vi "MainVI.vi"() -> ()   [LabVIEW 2020]
panel:
  in  "VOLUME (L)":dbl
  in  "FILL":bool
  in  "SET":bool
  in  "RE":bool
  in  "Down R":bool
  in  "R-L":bool
  in  "Up":bool
  in  "Hold":bool
  in  "Down":bool
  out "Boolean":bool
  out "Tank":dbl(slide) scale=0.0..100.0
  out "Boolean 2":bool
  # "EXTENDED BOTTLE SHIFTER"
  # "KUNAL KUMAR CHOUHAN"
  # "MALAVIYA NATIONAL INSTITUTE OF TECHNOLOGY"
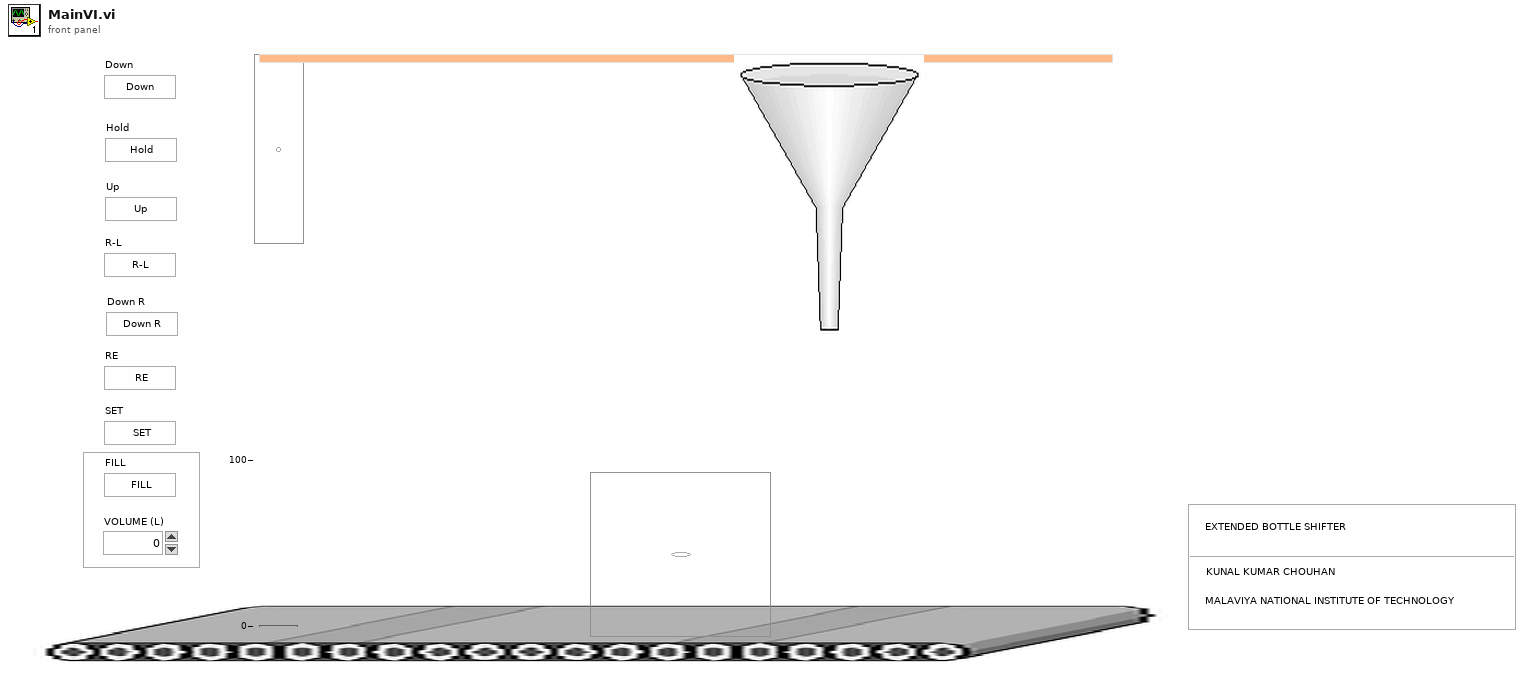
[diagram p1: front panel]
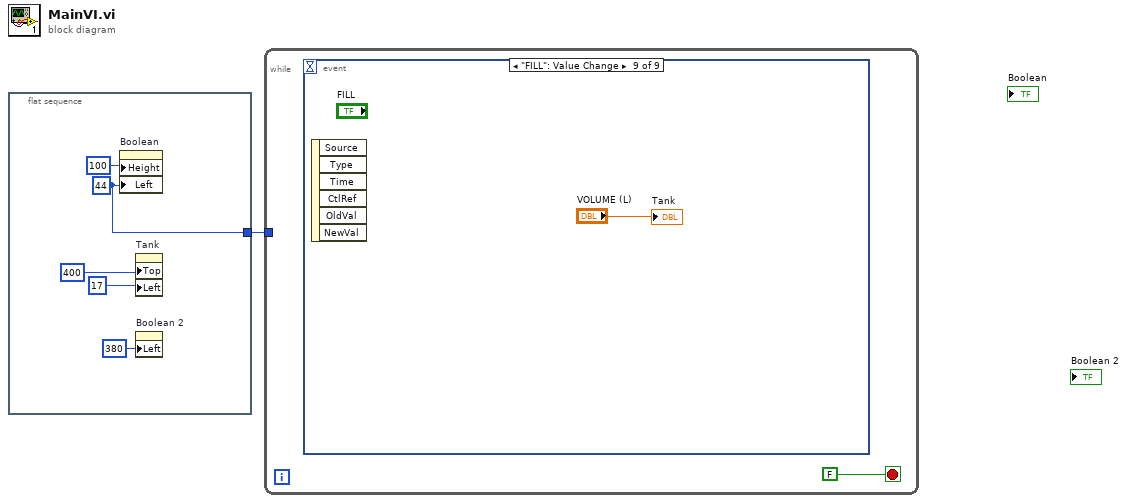
[diagram p0: block diagram]
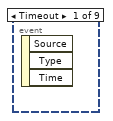
[diagram p2: hidden frame]
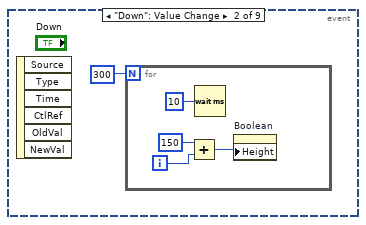
[diagram p3: hidden frame]
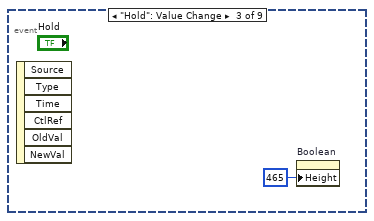
[diagram p4: hidden frame]
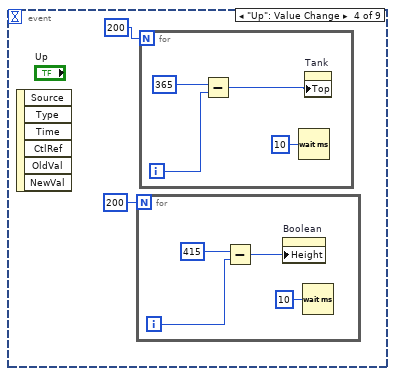
[diagram p5: hidden frame]
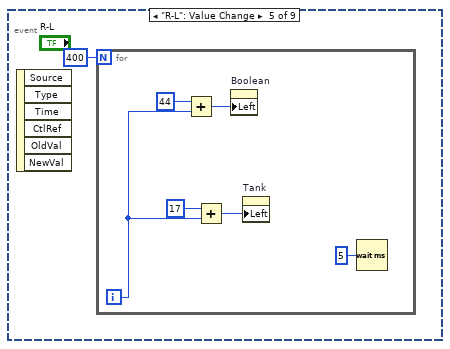
[diagram p6: hidden frame]
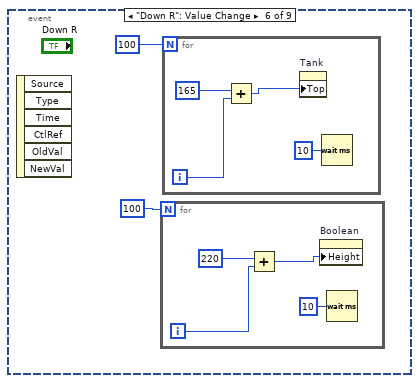
[diagram p7: hidden frame]
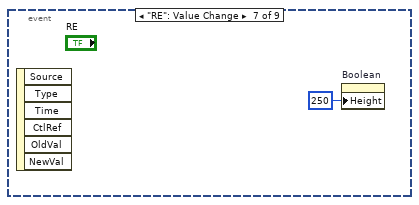
[diagram p8: hidden frame]
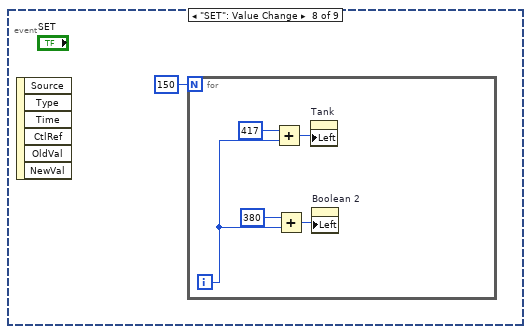
[diagram p9: hidden frame]
diagram:
  n1 = flat-sequence {
    tunnel: [w5] -> w1
    frame #0 {
      w5 = 44 ("Position:Left")
      n2 = property on="Boolean" class="Bool (strict)"("Height"=u32 100 ("Button Size:Height"), "Left"=w5) -> ()  [unwired: 2 in, 2 out]
      n3 = property on="Tank" class="Slide (strict)"("Top"=400 ("Position:Top"), "Left"=17 ("Position:Left")) -> ()  [unwired: 2 in, 2 out]
      n4 = property on="Boolean 2" class="Bool (strict)"("Left"=380 ("Position:Left")) -> ()  [unwired: 2 in, 2 out]
    }
  }
  n5 = while {
    tunnel: w1 -> [_]
    stop <- FALSE stop-if-true
    n6 = event shown="[8] \"FILL\": Value Change" {
      selector: _ -> [_ _ _ _ _ _ _ _ _]
      dyn-events: _ -> [_ _ _ _ _ _ _ _ _]
      timeout: _ -> [_ _ _ _ _ _ _ _ _]
      event Timeout {
        n7 = event-data() -> ()  [unwired: 1 in, 3 out]
      }
      event "Down": Value Change {
        n8 = event-data() -> ()  [unwired: 1 in, 6 out]
        n9 = for {
          N: 300 -> [_]
          i -> [w10]
          n10 = Add(x=150, y=w10) -> (x+y=w9:i32)
          n11 = Wait (ms)(milliseconds to wait=u32 10) -> ()  [unwired: 1 out]
          n12 = property on="Boolean" class="Bool (strict)"("Height"=w9) -> ()  [unwired: 2 in, 2 out]
        }
      }
      event "Hold": Value Change {
        n13 = event-data() -> ()  [unwired: 1 in, 6 out]
        n14 = property on="Boolean" class="Bool (strict)"("Height"=u32 465 ("Button Size:Height")) -> ()  [unwired: 2 in, 2 out]
      }
      event "Up": Value Change {
        n15 = event-data() -> ()  [unwired: 1 in, 6 out]
        n16 = for {
          N: 200 -> [_]
          i -> [w18]
          n17 = Subtract(x=415, y=w18) -> (x-y=w16:i32)
          n18 = property on="Boolean" class="Bool (strict)"("Height"=w16) -> ()  [unwired: 2 in, 2 out]
          n19 = Wait (ms)(milliseconds to wait=u32 10) -> ()  [unwired: 1 out]
        }
        n20 = for {
          N: 200 -> [_]
          i -> [w22]
          n21 = Subtract(x=365, y=w22) -> (x-y=w20:i32)
          n22 = Wait (ms)(milliseconds to wait=u32 10) -> ()  [unwired: 1 out]
          n23 = property on="Tank" class="Slide (strict)"("Top"=w20) -> ()  [unwired: 2 in, 2 out]
        }
      }
      event "R-L": Value Change {
        n24 = event-data() -> ()  [unwired: 1 in, 6 out]
        n25 = for {
          N: 400 -> [_]
          i -> [w29]
          n26 = Add(x=44, y=w29) -> (x+y=w30:i32)
          n27 = Add(x=17, y=w29) -> (x+y=w25:i32)
          n28 = property on="Boolean" class="Bool (strict)"("Left"=w30) -> ()  [unwired: 2 in, 2 out]
          n29 = property on="Tank" class="Slide (strict)"("Left"=w25) -> ()  [unwired: 2 in, 2 out]
          n30 = Wait (ms)(milliseconds to wait=u32 5) -> ()  [unwired: 1 out]
        }
      }
      event "Down R": Value Change {
        n31 = event-data() -> ()  [unwired: 1 in, 6 out]
        n32 = for {
          N: 100 -> [_]
          i -> [w35]
          n33 = Add(x=220, y=w35) -> (x+y=w33:i32)
          n34 = property on="Boolean" class="Bool (strict)"("Height"=w33) -> ()  [unwired: 2 in, 2 out]
          n35 = Wait (ms)(milliseconds to wait=u32 10) -> ()  [unwired: 1 out]
        }
        n36 = for {
          N: 100 -> [_]
          i -> [w39]
          n37 = Add(x=165, y=w39) -> (x+y=w37:i32)
          n38 = property on="Tank" class="Slide (strict)"("Top"=w37) -> ()  [unwired: 2 in, 2 out]
          n39 = Wait (ms)(milliseconds to wait=u32 10) -> ()  [unwired: 1 out]
        }
      }
      event "RE": Value Change {
        n40 = event-data() -> ()  [unwired: 1 in, 6 out]
        n41 = property on="Boolean" class="Bool (strict)"("Height"=u32 250 ("Button Size:Height")) -> ()  [unwired: 2 in, 2 out]
      }
      event "SET": Value Change {
        n42 = event-data() -> ()  [unwired: 1 in, 6 out]
        n43 = for {
          N: 150 -> [_]
          i -> [w45]
          n44 = Add(x=417, y=w45) -> (x+y=w47:i32)
          n45 = Add(x=380, y=w45) -> (x+y=w46:i32)
          n46 = property on="Tank" class="Slide (strict)"("Left"=w47) -> ()  [unwired: 2 in, 2 out]
          n47 = property on="Boolean 2" class="Bool (strict)"("Left"=w46) -> ()  [unwired: 2 in, 2 out]
        }
      }
      event "FILL": Value Change {
        n48 = event-data() -> ()  [unwired: 1 in, 6 out]
        "Tank" <- "VOLUME (L)"
      }
    }
  }
